vi "h5_2D_U16_stacking.vi"(5 "max_repeats":i32=-1, 6 "Attributes":variant, 7 "TYPE":string="IMG", 8 "error in (no error)":errorcluster, 9 "2D U16":u16[][](array[numeric]), 10 "SQUID":string="1", 11 "H5":path[](array[path])) -> (0 "error out":errorcluster, 2 "Exists":bool)   [LabVIEW 2013]
uses:
  <vilib>/addons/h5labview2/file/H5Fmode.ctl
  <vilib>/addons/h5labview2/base/lib_path.vi
  <vilib>/addons/h5labview2/base/H5Equery.vi
  <vilib>/addons/h5labview2/dataset/H5Dwrite.llb/H5Dwrite.xnode
  <vilib>/addons/h5labview2/base/hid_t.ctl
  <vilib>/addons/h5labview2/file/H5F.lvlib
  <vilib>/addons/h5labview2/group/H5G.lvlib
  <vilib>/addons/h5labview2/dataset/H5D.lvlib
  <vilib>/addons/h5labview2/attrib/H5A.lvlib
  <vilib>/addons/h5labview2/space/H5S.lvlib
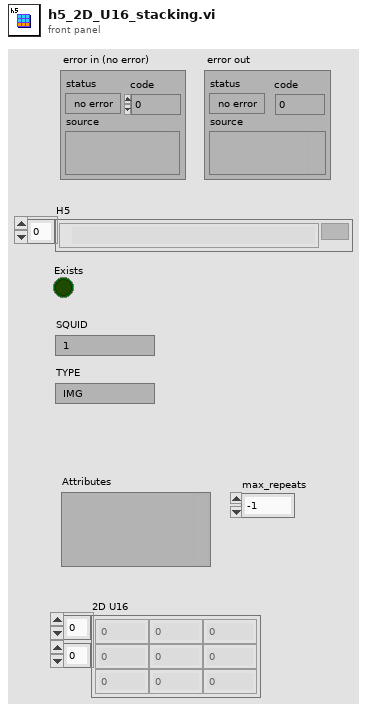
[diagram p1: front panel]
types:
  T1 = typedef "Semaphore RefNum" = refnum<k1>
  T2 = typedef "H5F.lvlib/H5Fmode.ctl" = enum16{"read-only", "read-write", "overwrite", "create new", "open or create"}
  T3 = typedef "hid_t.ctl" = i32
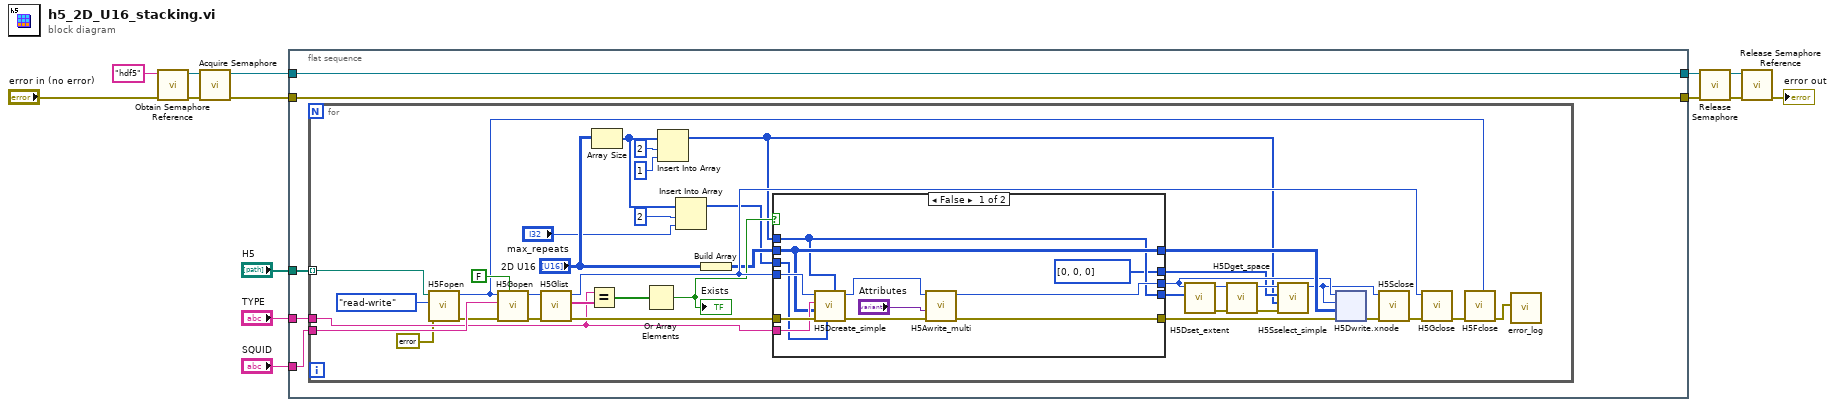
[diagram p0: block diagram]
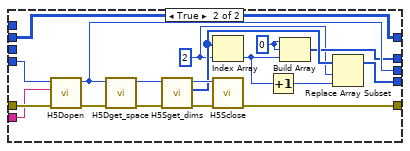
[diagram p2: hidden frame]
diagram:
  n1 = call <vilib>:"Obtain Semaphore Reference.vi"("error in (no error)"="error in (no error)", "name (unnamed)"="hdf5") -> ("error out"=w13:errorcluster, "semaphore"=w14:T1)  [unwired: 3 in, 1 out]
  n2 = call <vilib>:"Acquire Semaphore.vi"("error in (no error)"=w13, "semaphore"=w14) -> ("error out"=w7:errorcluster, "semaphore out"=w6:T1)  [unwired: 3 in, 1 out]
  n3 = flat-sequence {
    tunnel: [w19] -> w8
    tunnel: w7 -> [w19]
    tunnel: w6 -> [w18]
    tunnel: [w18] -> w5
    tunnel: "H5" -> [w17]
    tunnel: "SQUID" -> [w16]
    tunnel: "TYPE" -> [w15]
    frame #0 {
      n4 = for {
        tunnel: w17 -> [w50] mode=indexing
        tunnel: w16 -> [w51]
        tunnel: w15 -> [w42]
        n5 = call <vilib>:"H5Fopen.vi"("error in (no error)"=errorcluster {"status"=FALSE, "code"=0, "source"=""}, "mode (read-only)"=H5Fmode."read-write", "path"=w50) -> ("error out"=w49:errorcluster, "ref out"=w48:T3)  [unwired: 7 in]
        n6 = call <vilib>:"H5Gopen.vi"("create? (F)"=FALSE, "error in (no error)"=w49, "name"=w51, "ref in"=w48) -> ("error out"=w46:errorcluster, "group out"=w47:T3)  [unwired: 6 in]
        n7 = call <vilib>:"H5Glist.vi"("error in (no error)"=w46, "ref in"=w47) -> ("error out"=w45:errorcluster, "names"=w43:string[], "ref out"=w44:T3)  [unwired: 6 in, 1 out]
        n8 = Equal?(x=w42, y=w43) -> (x = y?=w41:bool[])
        n9 = Array Size(array="2D U16") -> (size(s)=w34:i32[])
        n10 = Or Array Elements(Boolean array=w41) -> (logical OR=w40:bool)
        "Exists" <- w40
        n11 = Insert Into Array(array=w34, index=2, new element=1 ("new element/subarray")) -> (w23:i32[])
        n12 = Insert Into Array(array=w34, index=2, new element="max_repeats") -> (w31:i32[])
        n13 = Build Array("2D U16") -> (w36:u16[][][])
        n14 = case shown="False" w40 {
          tunnel: w45 -> [w87 w104]
          tunnel: w36 -> [w84 w105]
          tunnel: w44 -> [w86 w102]
          tunnel: w42 -> [w85 w103]
          tunnel: [w78 w97] -> w35
          tunnel: w23 -> [w77 _]
          tunnel: [w84 w105] -> w55
          tunnel: [w79 w95] -> w26
          tunnel: w31 -> [w80 _]
          tunnel: [w77 w92] -> w25
          tunnel: [u64[] [0, 0, 0] ("start") w89] -> w24
          frame False {
            n15 = call <vilib>:"H5Dcreate_simple.vi"("chunk size"=w77, "initial size"=w80, "error in (no error)"=w87, "type in"=w84, "name"=w85, "ref in"=w86) -> ("error out"=w82:errorcluster, "dset out"=w81:T3)  [unwired: 4 in]
            n16 = call <vilib>:"H5Awrite_multi.vi"("error in (no error)"=w82, "variant in"="Attributes", "ref in"=w81) -> ("error out"=w78:errorcluster, "ref out"=w79:T3)  [unwired: 7 in]
          }
          frame True {
            w90 = u64 0 ("element")
            w88 = 2 ("index")
            n17 = call <vilib>:"H5Dopen.vi"("error in (no error)"=w104, "name"=w103, "loc in"=w102) -> ("error out"=w96:errorcluster, "dset out"=w95:T3)  [unwired: 7 in]
            n18 = call <vilib>:"H5Dget_space.vi"("error in (no error)"=w96, "ref in"=w95) -> ("error out"=w101:errorcluster, "space out"=w100:T3)  [unwired: 8 in]
            n19 = call <vilib>:"H5Sget_dims.vi"("error in (no error)"=w101, "space in"=w100) -> ("error out"=w99:errorcluster, "dims"=w93:u32[], "space out"=w98:T3)  [unwired: 6 in, 1 out]
            n20 = Index Array(array=w93, index=w88) -> (element=w91:u32)
            n21 = call <vilib>:"H5Sclose.vi"("error in (no error)"=w99, "space in"=w98) -> ("error out"=w97:errorcluster)  [unwired: 9 in]
            n22 = Increment(x=w91) -> (x+1=w94:u32)
            n23 = Build Array(w90, w90, w91) -> (w89:u64[])
            n24 = Replace Array Subset(array=w93, new element=w94, index=w88) -> (w92:u32[])
          }
        }
        n25 = call <vilib>:"H5Dset_extent.vi"("new size"=w25, "dset in"=w26) -> ("error out"=w30:errorcluster, "dset out"=w29:T3)  [unwired: 8 in]
        n26 = call <vilib>:"H5Dget_space.vi"("error in (no error)"=w30, "ref in"=w29) -> ("error out"=w28:errorcluster, "space out"=w27:T3)  [unwired: 8 in]
        n27 = call <vilib>:"H5Sselect_simple.vi"("error in (no error)"=w28, "count"=w23, "start"=w24, "space in"=w27) -> ("space out"=w22:T3)  [unwired: 6 in, 1 out]
        n28 = xnode "H5Dwrite.xnode"("error in (no error)"=w35, "data"=w55, "file space"=w22, "ref in"=w26) -> ("error out"=w56:errorcluster)  [unwired: 3 in, 2 out]
        n29 = call <vilib>:"H5Sclose.vi"("error in (no error)"=w56, "space in"=w22) -> ("error out"=w54:errorcluster)  [unwired: 9 in]
        n30 = call <vilib>:"H5Gclose.vi"("error in (no error)"=w54, "group in"=w44) -> ("error out"=w52:errorcluster)  [unwired: 9 in]
        n31 = call <vilib>:"H5Fclose.vi"("error in (no error)"=w52, "ref"=w48) -> ("error out"=w20:errorcluster)  [unwired: 9 in]
        n32 = call "error_log.vi"("error"=w20) -> ()  [unwired: 10 in]
      }
    }
  }
  n33 = call <vilib>:"Release Semaphore.vi"("error in (no error)"=w8, "semaphore"=w5) -> ("error out"=w9:errorcluster, "semaphore out"=w10:T1)  [unwired: 4 in]
  n34 = call <vilib>:"Release Semaphore Reference.vi"("error in (no error)"=w9, "semaphore"=w10) -> ("error out"=→"error out":errorcluster)  [unwired: 8 in, 1 out]
